vi "Destroy.vi"(0 "reference in":refnum<class "WaveFile.lvclass">, 5 "error in (no error)":errorcluster) -> (14 "reference out":refnum<class "WaveFile.lvclass">, 19 "error out":errorcluster)   [LabVIEW 2020, in "WaveFile.lvclass"]
doc: "Destructor."
uses:
  WaveFile.lvclass
  API/Generic Utilities_class/Generic Utilities.lvclass
  API/GSwFormDSP_class/GSwFormDSP.lvclass
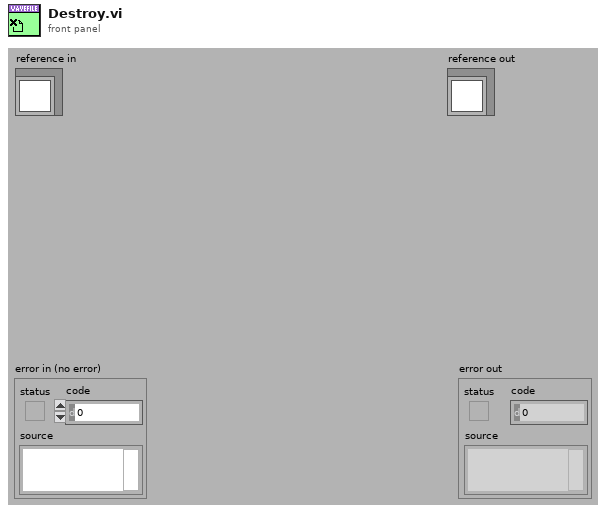
[diagram p1: front panel]
types:
  T1 = typedef "WaveFile.lvclass/ObjectAttributes.ctl" = cluster{"Time Data":refnum<class "GSwFormDSP.lvclass">, "New Time Data Obj?":bool, "NIST File Header":T2}
  T2 = typedef "WaveFile.lvclass/NIST File Header.ctl" = cluster{"Version":string, "Header Nb Bytes":i32, "Nb Samples":i32, "Nb Bytes/sample":i32, "Nb Channels":i32, "byte order":enum16{"big-endian, network order", "native, host order", "little-endian"}, "Fs":dbl, "Valid Header?":bool}
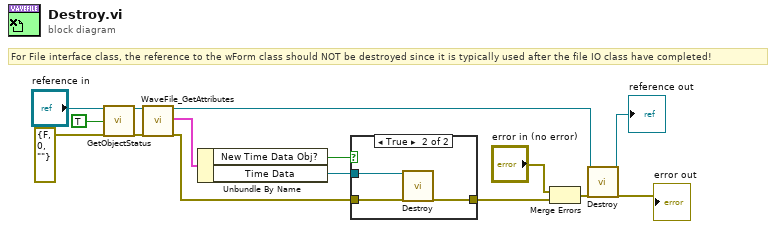
[diagram p0: block diagram]
diagram:
  # "For File interface class, the reference to the wForm class should NOT be destroyed since it is typically used after the file IO class have completed!"
  n1 = call-dynamic "GetObjectStatus.vi"("reference in"="reference in", "simple info (F)"=TRUE ("simple info"), "error in (no error)"=errorcluster {"status"=FALSE, "code"=0, "source"=""}) -> ("reference out"=w8:refnum<class "WaveFile.lvclass">, "error out"=w6:errorcluster)  [unwired: 5 in, 10 out]
  n2 = call "WaveFile_GetAttributes.vi"("reference in"=w8, "error in (no error)"=w6) -> ("reference out"=w7:refnum<class "WaveFile.lvclass">, "attributes"=w1:T1, "error out"=w3:errorcluster)  [unwired: 14 in, 1 out]
  n3 = Unbundle By Name(w1) -> ("New Time Data Obj?"=w4:bool, "Time Data"=w5:refnum<class "GSwFormDSP.lvclass">)
  n4 = case shown="True" w4 {
    tunnel: w5 -> [_ w19]
    tunnel: w3 -> [w16 w18]
    tunnel: [w16 w17] -> w2
    frame False {
    }
    frame True {
      n5 = call-dynamic "Destroy.vi"("reference in"=w19, "error in (no error)"=w18) -> ("error out"=w17:errorcluster)  [unwired: 16 in, 1 out]
    }
  }
  n6 = Merge Errors("error in (no error)", w2) -> (w14:errorcluster)
  n7 = call-parent "Destroy.vi"("reference in"=w7, "error in (no error)"=w14) -> ("reference out"=→"reference out":refnum<class "WaveFile.lvclass">, "error out"=→"error out":errorcluster)  [unwired: 16 in]
